vi "niRFSysCalReader Interpolate Variant Name.vi"() -> (3 "Interpolation State Name":string)   [LabVIEW 2017, in "niRFSysCalReader.lvlib"]
uses:
  niRFSysCalReader.lvlib
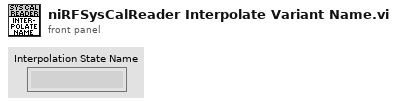
[diagram p1: front panel]
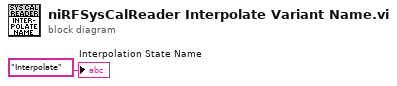
[diagram p0: block diagram]
diagram:
  "Interpolation State Name" <- "Interpolate" ("name")
